vi "Configuration Dialog Box.vi"(8 "error in (no error)":errorcluster, 11 "Configuration Settings In":T2={"Offset"=0.0, "Signal Type"=enum."Sine Wave", "Frequency"=10.0, "Amplitude"=1.0, "Phase"=0.0, "Noise Amplitude"=1.0} {"Noise Amplitude" format="%.2p"; "Phase" format="%.2p"; "Amplitude" format="%0.2p"; "Frequency" format="%0.2p"; "Offset" format="%0.2p"}) -> (0 "error out":errorcluster, 3 "Configuration Settings Out":T2={"Offset"=0.0, "Signal Type"=enum."Sine Wave", "Frequency"=10.0, "Amplitude"=1.0, "Phase"=0.0, "Noise Amplitude"=1.0} {"Noise Amplitude" format="%.2p"; "Phase" format="%.2p"; "Amplitude" format="%0.2p"; "Frequency" format="%0.2p"; "Offset" format="%0.2p"})   [LabVIEW 2015]
uses:
  controls/Configuration Settings.ctl
panel:
  in  "Noise Amplitude":dbl=1.0 format="%.2p"
  in  "Phase":dbl format="%.2p"
  in  "Amplitude":dbl=1.0 format="%0.2p"
  in  "Frequency":dbl=10.0 format="%0.2p"
  in  "Signal Type":T1(ring)
  in  "Offset":dbl format="%0.2p"
  in  "Cancel":bool
  in  "Ok":bool
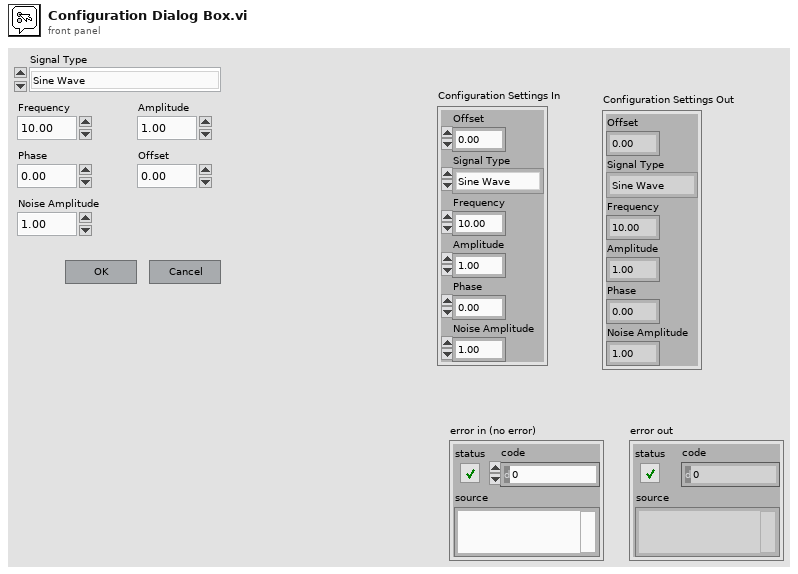
[diagram p1: front panel]
types:
  T1 = enum16{"Sine Wave", "Triangle Wave", "Square Wave", "Sawtooth Wave"}
  T2 = typedef "Configuration Settings.ctl" = cluster{"Offset":dbl, "Signal Type":enum16{"Sine Wave", "Triangle Wave", "Square Wave", "Sawtooth Wave"}, "Frequency":dbl, "Amplitude":dbl, "Phase":dbl, "Noise Amplitude":dbl}
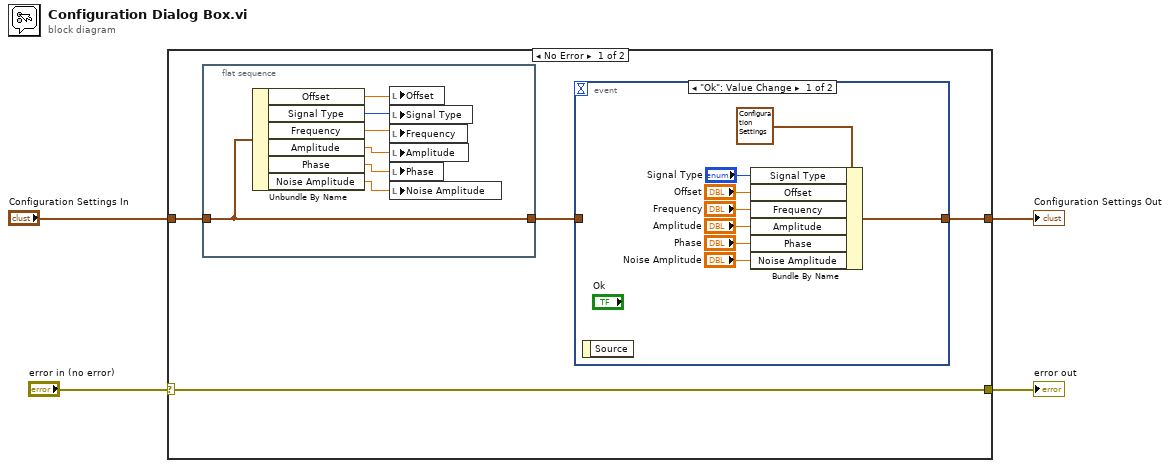
[diagram p0: block diagram]
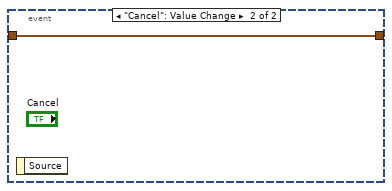
[diagram p2: hidden frame]
diagram:
  n1 = case shown="No Error" "error in (no error)" {
    selector: "error in (no error)" -> [w8 w26]
    tunnel: [w8 w26] -> w3
    tunnel: "Configuration Settings In" -> [w6 w25]
    tunnel: [w7 w25] -> w1
    frame No Error {
      n2 = flat-sequence {
        tunnel: w6 -> [w9]
        tunnel: [w9] -> w5
        frame #0 {
          n3 = Unbundle By Name(w9) -> ("Offset"=w15:dbl, "Signal Type"=w14:T1, "Frequency"=w13:dbl, "Amplitude"=w12:dbl, "Phase"=w11:dbl, "Noise Amplitude"=w10:dbl)
          n4 = local write "Offset"(w15) -> ()
          n5 = local write "Signal Type"(w14) -> ()
          n6 = local write "Frequency"(w13) -> ()
          n7 = local write "Amplitude"(w12) -> ()
          n8 = local write "Phase"(w11) -> ()
          n9 = local write "Noise Amplitude"(w10) -> ()
        }
      }
      n10 = event shown="[0] \"Ok\": Value Change" {
        selector: _ -> [_ _]
        dyn-events: _ -> [_ _]
        timeout: _ -> [_ _]
        tunnel: [w16 w24] -> w7
        tunnel: w5 -> [_ w24]
        event "Ok": Value Change {
          n11 = event-data() -> ()  [unwired: 1 in, 1 out]
          n12 = Bundle By Name(cluster=T2 {"Offset"=0.0, "Signal Type"=enum."Sine Wave", "Frequency"=10.0, "Amplitude"=1.0, "Phase"=0.0, "Noise Amplitude"=1.0} ("Configuration Settings Out"), "Signal Type"="Signal Type", "Offset"="Offset", "Frequency"="Frequency", "Amplitude"="Amplitude", "Phase"="Phase", "Noise Amplitude"="Noise Amplitude") -> (w16:T2)
        }
        event "Cancel": Value Change {
          n13 = event-data() -> ()  [unwired: 1 in, 1 out]
        }
      }
    }
    frame Error {
    }
  }
  "Configuration Settings Out" <- w1
  "error out" <- w3
